vi "PIEZO_main.vi"() -> ()   [LabVIEW 2015]
uses:
  CONTROLS/Q_MCL_piezo_element.ctl
  CONTROLS/Q_main_element.ctl
  GLOBAL/Global_MCL_piezo.vi
  GLOBAL/Global_ABORT.vi
  GLOBAL/Global_MAIN.vi
  <vilib>/Utility/inputDevices.llb/keyboardAcquire.vi
  <vilib>/Utility/inputDevices.llb/closeKeyboard.vi
  <userlib>/Madlib.dll
  <vilib>/addons/control/pid/NI_PID_autopid.lvlib
panel:
  in  "Q_MCL_Piezo":T1
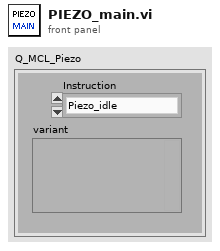
[diagram p1: front panel]
types:
  T1 = typedef "Q_MCL_piezo_element.ctl" = cluster{"variant":variant, "Instruction":enum16{"Piezo_idle", "Piezo_initialize", "Piezo_error", "Piezo_security_stop", "Piezo_read_z", "Piezo_move_z", "Piezo_keyboard_move", "Piezo_close_autofocus_calibration_ramp", "Piezo_change_init_state", "Piezo_init_autofocus", "Piezo_init_autofocus_merFISH_TL", "Piezo_autofocus", "Piezo_autofocus_merFISH_TL", "Piezo_stop_autofocus", "Piezo_stop_autofocus_merFISH_TL", "Piezo_autofocus_lost", "Piezo_resume_autofocus_merFISH_TL", "Piezo_check_z_position_merFISH_TL", "Piezo_init_ramp", "Piezo_move_z_ramp", "Piezo_close_ramp", "Piezo_close_merFISH", "Piezo_stop"}}
  T2 = cluster{"Setpoint":dbl, "Ref channel":bool, "dimension size":i32, "X_derivation":dbl[], "Y_derivation":dbl[], "Slope":dbl, "iteration":i32, "PID gains":cluster{"proportional gain (Kc)":dbl, "integral time (Ti, min)":dbl, "derivative time (Td, min)":dbl}, "z0":dbl, "Switch":bool, "Autocalibration":bool, "Init":bool, "i IR lost":i32, "Derivation array":dbl[], "QPDcount":u32}
  T3 = typedef "Q_main_element.ctl" = cluster{"variant":variant, "Instruction":enum16{"Main_idle", "Main_initialize", "Main_initialize_TDMS", "Main_initialize_Queue", "Main_error", "Main_DAQ_initialization_results", "Main_ASI_initialization_results", "Main_Piezo_initialization_results", "Main_Valve_initialization_results", "Main_Pump_initialization_results", "Main_CAMERA_initialization_results", "Main_FPGA_initialization_results", "Main_DAQ_error", "Main_ASI_error", "Main_Piezo_error", "Main_CAMERA_error", "Main_Valve_error", "Main_Pump_error", "Main_FPGA_error", "Main_start_acquiring", "Main_not_acquiring", "Main_acquiring", "Main_stop_acquiring", "Main_change_exposure", "Main_change_z_scan_parameters", "Main_define_ROI", "Main_define_mosaic", "Main_read_kinetic_time", "Main_cooler", "Main_read_temperature", "Main_save_XY", "Main_load_XY", "Main_discard_XY", "Main_move_to_XY", "Main_measure_QPD", "Main_autofocus_calibration", "Main_autofocus_initialization", "Main_autofocus_stop", "Main_save_PID", "Main_change_H_valve_position", "Main_two_way_valve", "Main_save_movie", "Main_init_single_scan", "Main_single_scan", "Main_stop_single_scan", "Main_merFISH_illumination_parameters", "Main_merFISH_buffer_probe_list", "Main_merFISH_injections_procedure", "Main_merFISH_save_setpoint", "Main_merFISH_DAPI_parameters", "Main_merFISH_Brightfield_parameters", "Main_merFISH_save_embryo_ROI", "Main_merFISH_init", "Main_merFISH_resume", "Main_merFISH_start_autofocus", "Main_merFISH_open_close_valve_merFISH", "Main_merFISH_open_close_valve_photobleaching", "Main_merFISH_hybridization", "Main_merFISH_move_to_ROI", "Main_merFISH_wait_stabilization", "Main_merFISH_move_to_REF", "Main_merFISH_scan", "Main_merFISH_photobleaching_injection", "Main_merFISH_photobleaching", "Main_merFISH_send_email", "Main_merFISH_close", "Main_STOP"}}
  T4 = enum16{"0", "1", "2", "3", "4", "5", "6", "7", "8", "9", "A", "B", "C", "D", "E", "F", "G", "H", "I", "J", "K", "L", "M", "N", "O", "P", "Q", "R", "S", "T", "U", "V", "W", "X", "Y", "Z", "F1", "F2", "F3", "F4", "F5", "F6", "F7", "F8", "F9", "F10", "F11", "F12", "F13", "F14", "F15", "ADD", "BACK", "BACKSLASH", "CAPITAL", "COMMA", "DECIMAL", "DELETE", "DIVIDE", "DOWN", "END", "EQUALS", "ESCAPE", "GRAVE (`)", "HOME", "INSERT", "LBRACKET", "LCONTROL", "LEFT", "L ALT", "LSHIFT", "LWIN", "MINUS", "MULTIPLY", "NEXT", "NUMLOCK", "NUMPAD_0", "NUMPAD_1", "NUMPAD_2", "NUMPAD_3", "NUMPAD_4", "NUMPAD_5", "NUMPAD_6", "NUMPAD_7", "NUMPAD_8", "NUMPAD_9", "PAUSE", "PERIOD", "PRIOR (PG UP)", "RBRACKET", "RCONTROL", "RETURN", "RIGHT", "R ALT", "RSHIFT", "RWIN", "SCROLL", "SEMICOLON", "SLASH", "SPACE", "SUBTRACT", "TAB", "UP", "ENTER (num pad)", "' (quote)"}
  T5 = cluster{"PID gains":cluster{"proportional gain (Kc)":dbl, "integral time (Ti, min)":dbl, "derivative time (Td, min)":dbl}, "QPD ref":cluster{"X":sgl, "Y":sgl, "SUM":sgl, "count":u32}}
  T6 = enum16{"Piezo_idle", "Piezo_initialize", "Piezo_error", "Piezo_security_stop", "Piezo_read_z", "Piezo_move_z", "Piezo_keyboard_move", "Piezo_close_autofocus_calibration_ramp", "Piezo_change_init_state", "Piezo_init_autofocus", "Piezo_init_autofocus_merFISH_TL", "Piezo_autofocus", "Piezo_autofocus_merFISH_TL", "Piezo_stop_autofocus", "Piezo_stop_autofocus_merFISH_TL", "Piezo_autofocus_lost", "Piezo_resume_autofocus_merFISH_TL", "Piezo_check_z_position_merFISH_TL", "Piezo_init_ramp", "Piezo_move_z_ramp", "Piezo_close_ramp", "Piezo_close_merFISH", "Piezo_stop"}
  T7 = enum16{"0", "1", "2", "3", "4", "5", "6", "7", "8", "9", "A", "B", "C", "D", "E", "F", "G", "H", "I", "J", "K", "L", "M", "N", "O", "P", "Q", "R", "S", "T", "U", "V", "W", "X", "Y", "Z", "F1", "F2", "F3", "F4", "F5", "F6", "F7", "F8", "F9", "F10", "F11", "F12", "F13", "F14", "F15", "ADD", "BACK", "BACKSLASH", "CAPITAL", "COMMA", "DECIMAL", "DELETE", "DIVIDE", "DOWN", "END", "EQUALS", "ESCAPE", "GRAVE (`)", "HOME", "INSERT", "LBRACKET", "LCONTROL", "LEFT", "L ALT", "LSHIFT", "LWIN", "MINUS", "MULTIPLY", "NEXT", "NUMLOCK", "NUMPAD_0", "NUMPAD_1", "NUMPAD_2", "NUMPAD_3", "NUMPAD_4", "NUMPAD_5", "NUMPAD_6", "NUMPAD_7", "NUMPAD_8", "NUMPAD_9", "PAUSE", "PERIOD", "PRIOR (PG UP)", "RBRACKET", "RCONTROL", "RETURN", "RIGHT", "R ALT", "RSHIFT", "RWIN", "SCROLL", "SEMICOLON", "SLASH", "SPACE", "SUBTRACT", "TAB", "UP", "ENTER (num pad)", "' (quote)"}[]
  T8 = cluster{"proportional gain (Kc)":dbl, "integral time (Ti, min)":dbl, "derivative time (Td, min)":dbl}
  T9 = cluster{"X":sgl, "Y":sgl, "SUM":sgl, "count":u32}
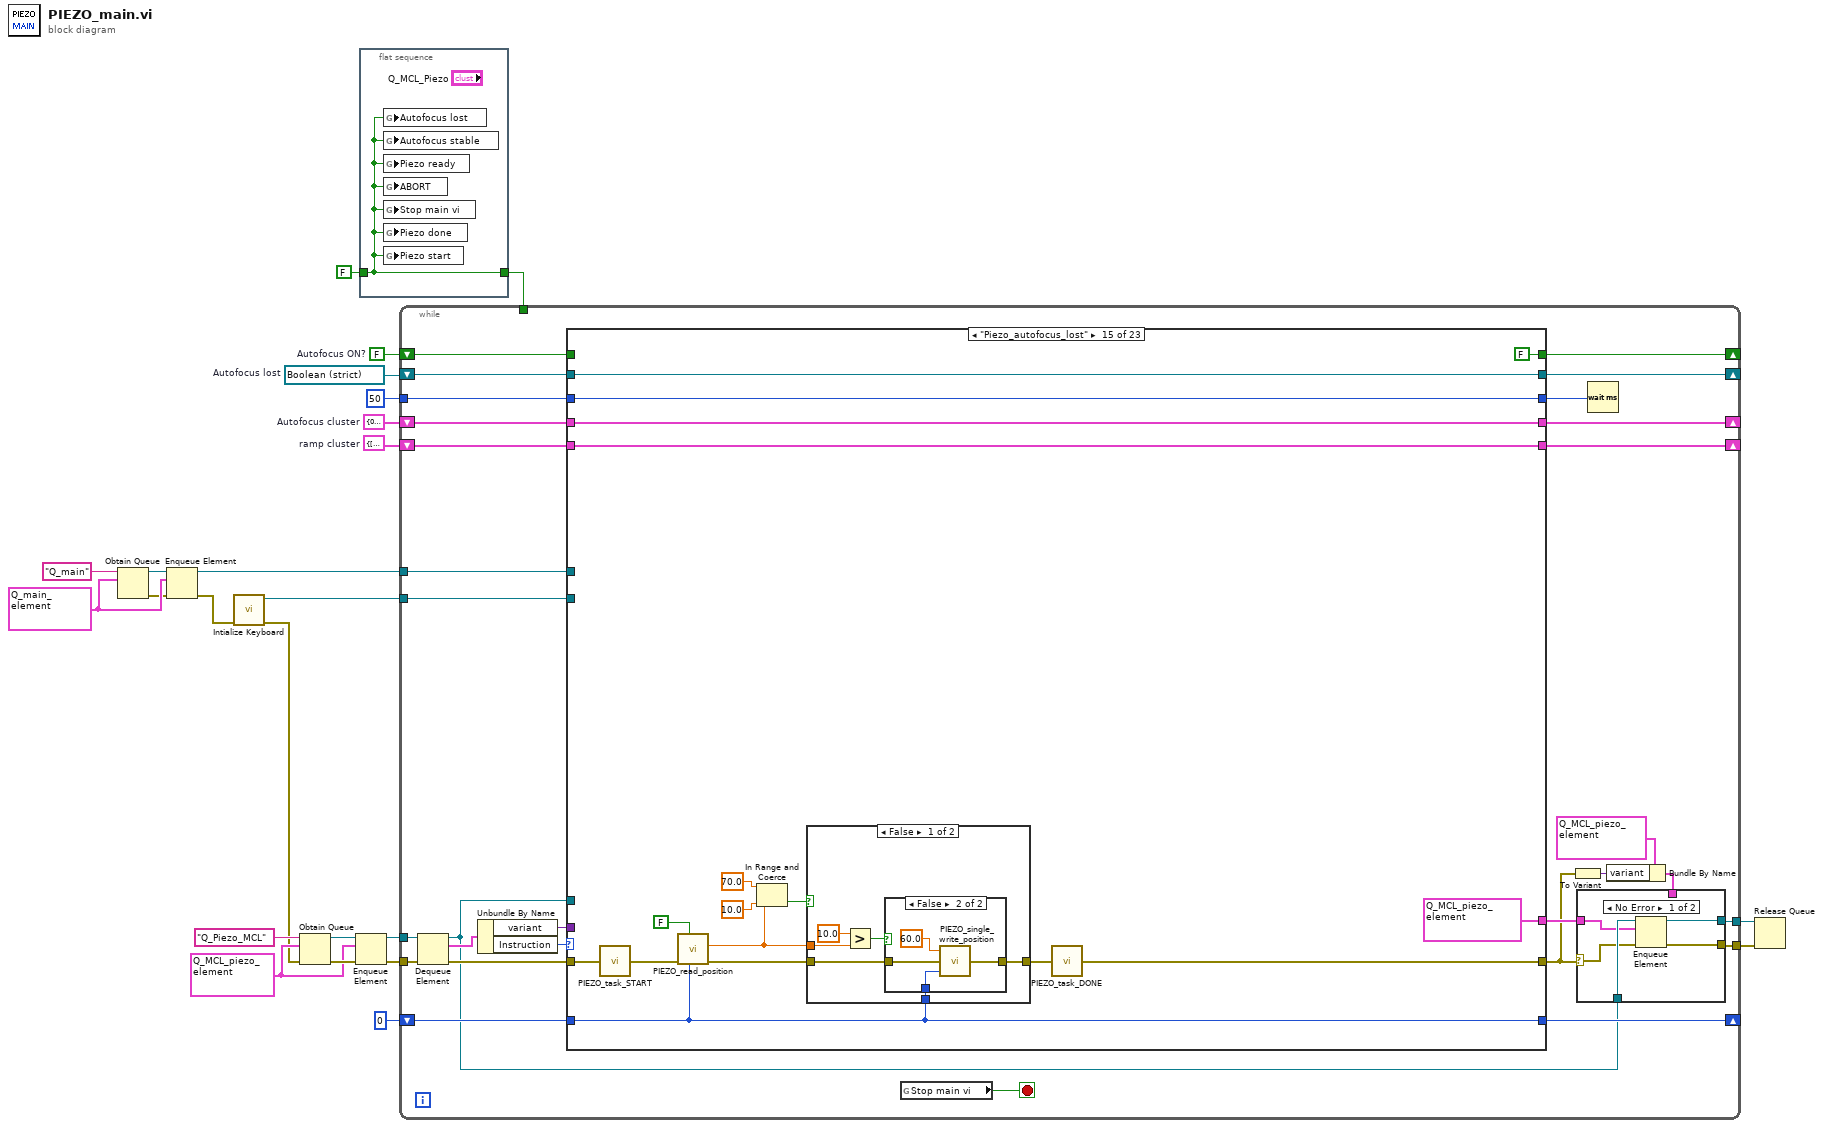
[diagram p0: block diagram]
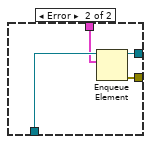
[diagram p2: hidden frame]
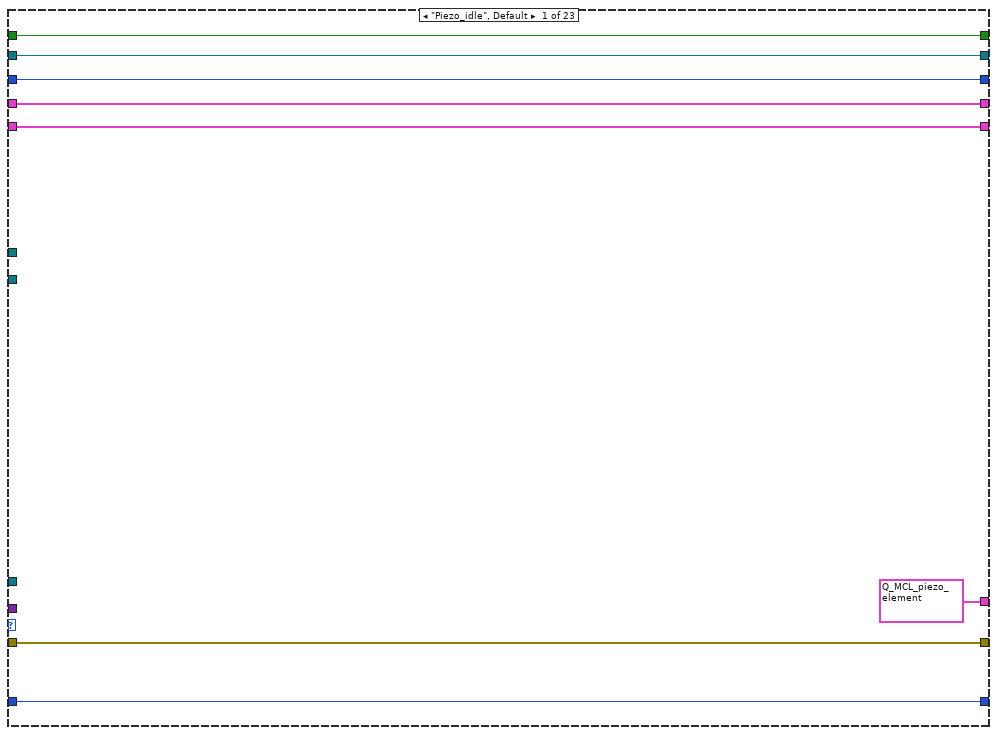
[diagram p3: hidden frame]
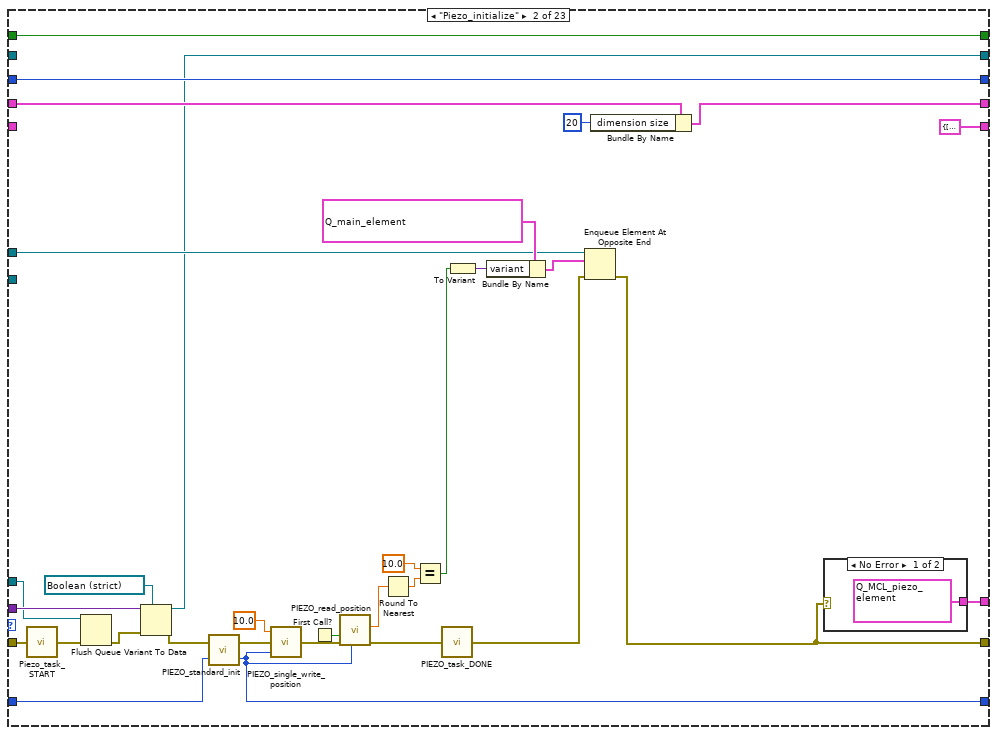
[diagram p4: hidden frame]
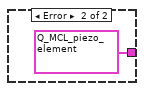
[diagram p5: hidden frame]
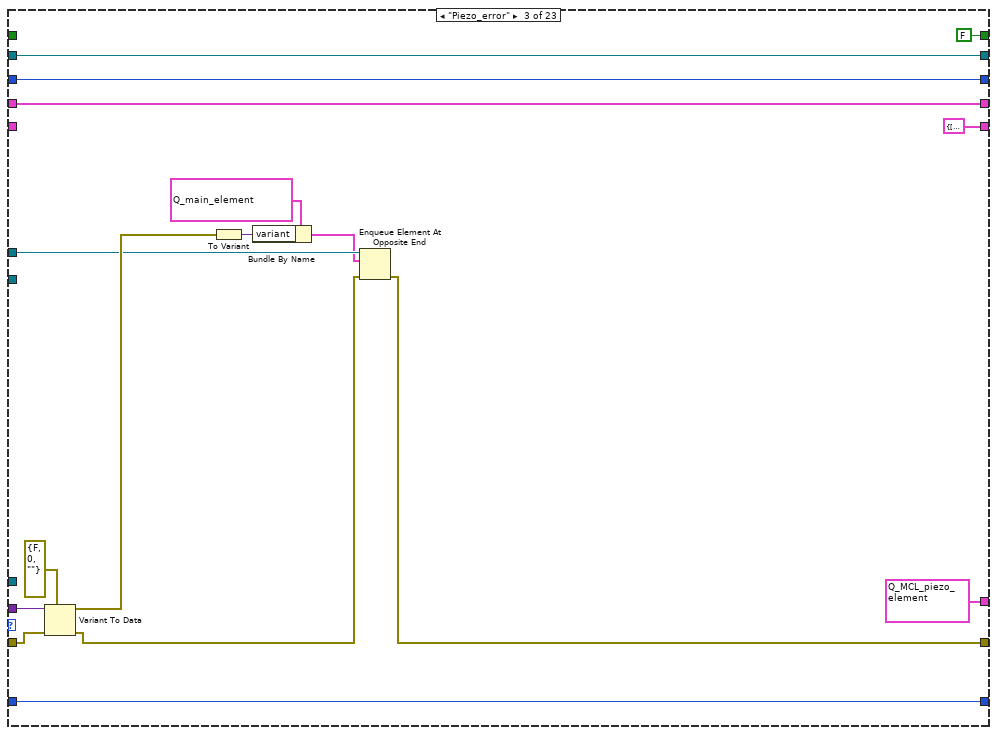
[diagram p6: hidden frame]
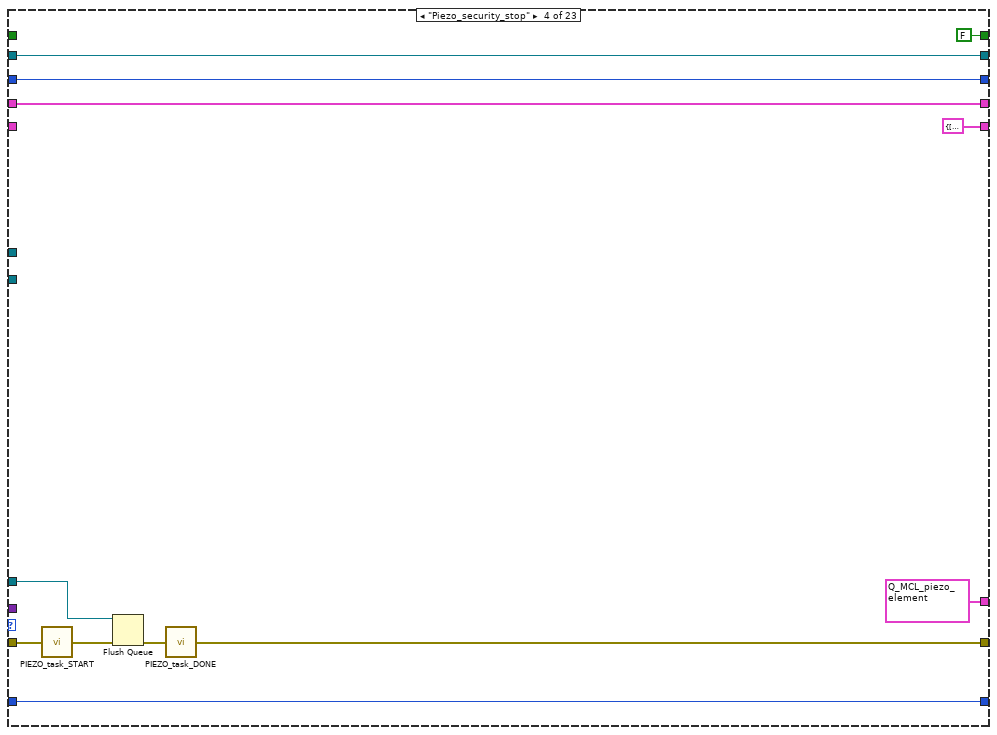
[diagram p7: hidden frame]
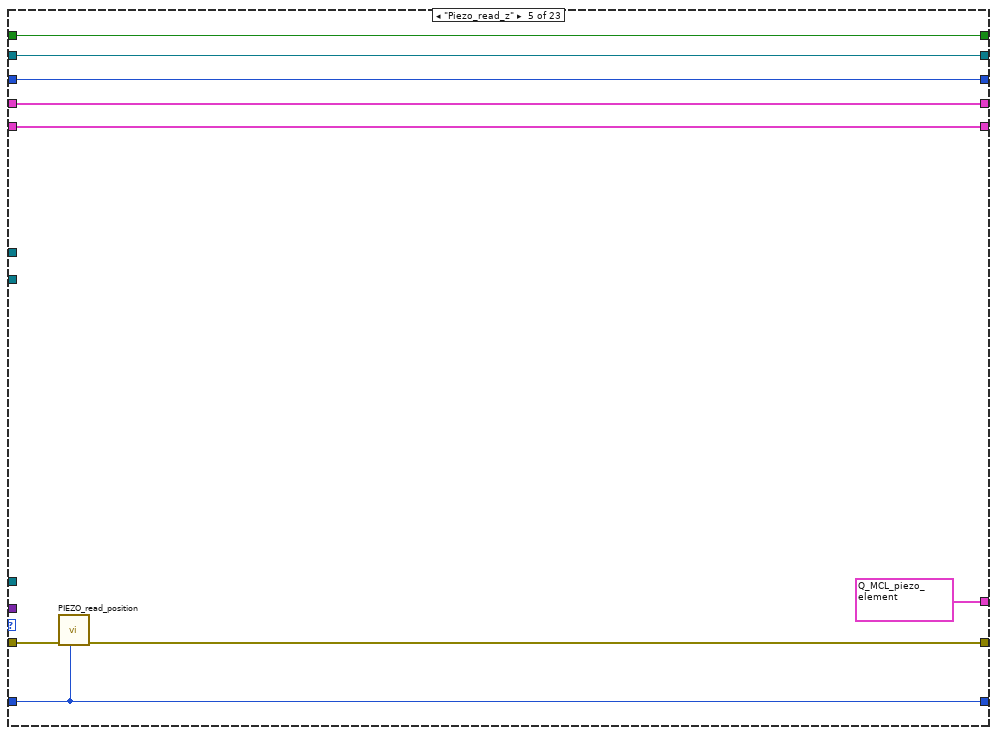
[diagram p8: hidden frame]
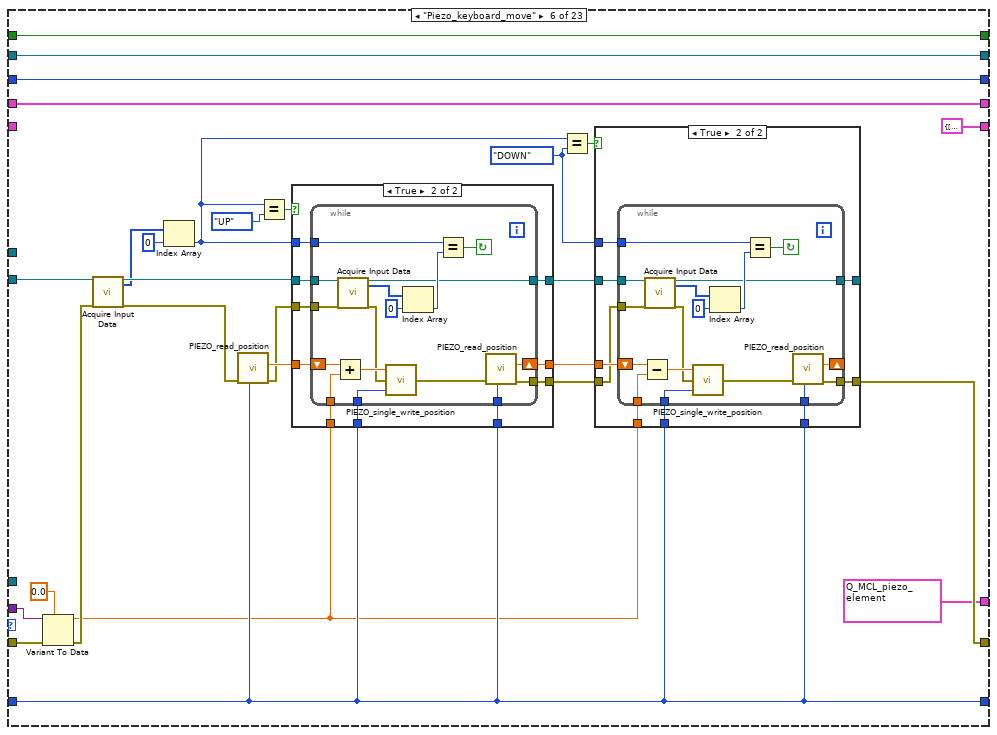
[diagram p9: hidden frame]
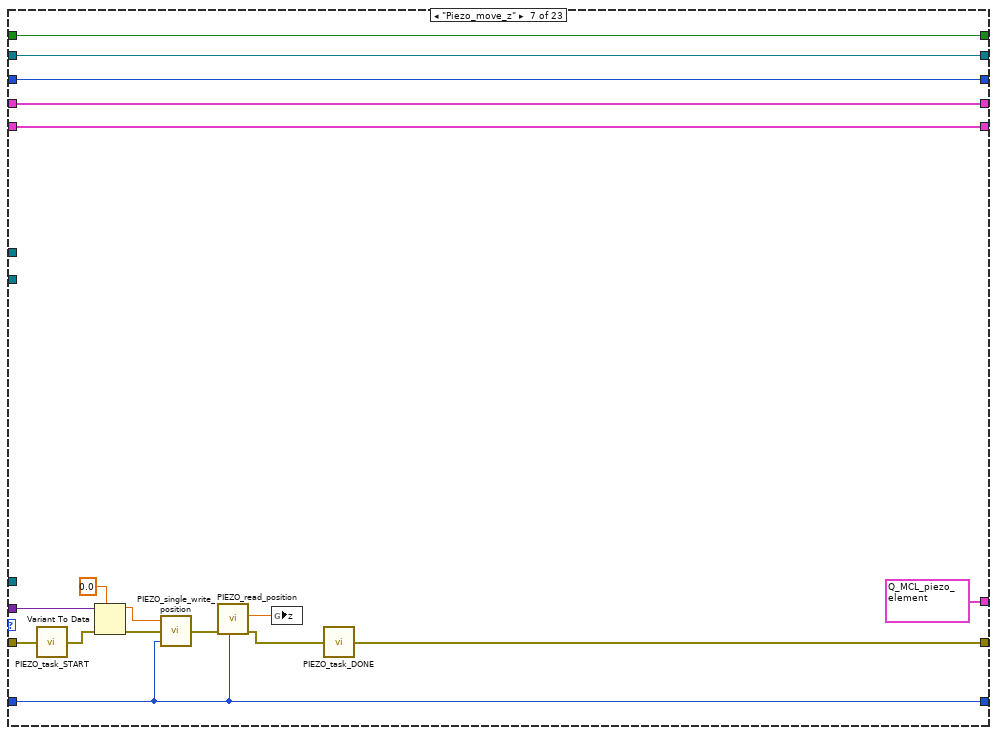
[diagram p12: hidden frame]
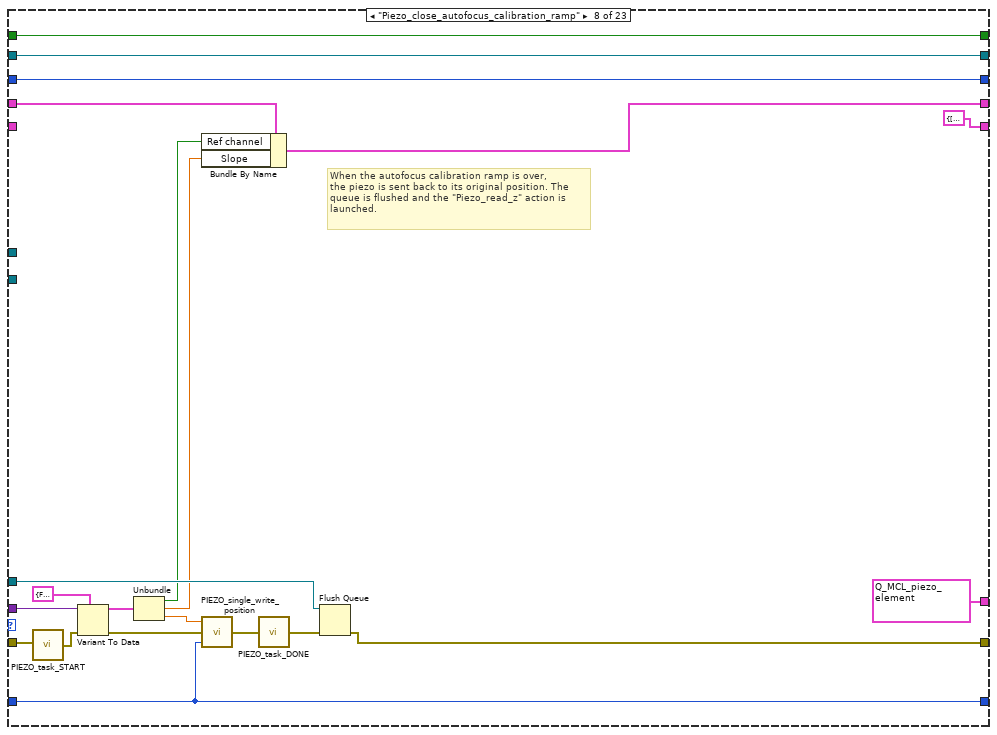
[diagram p13: hidden frame]
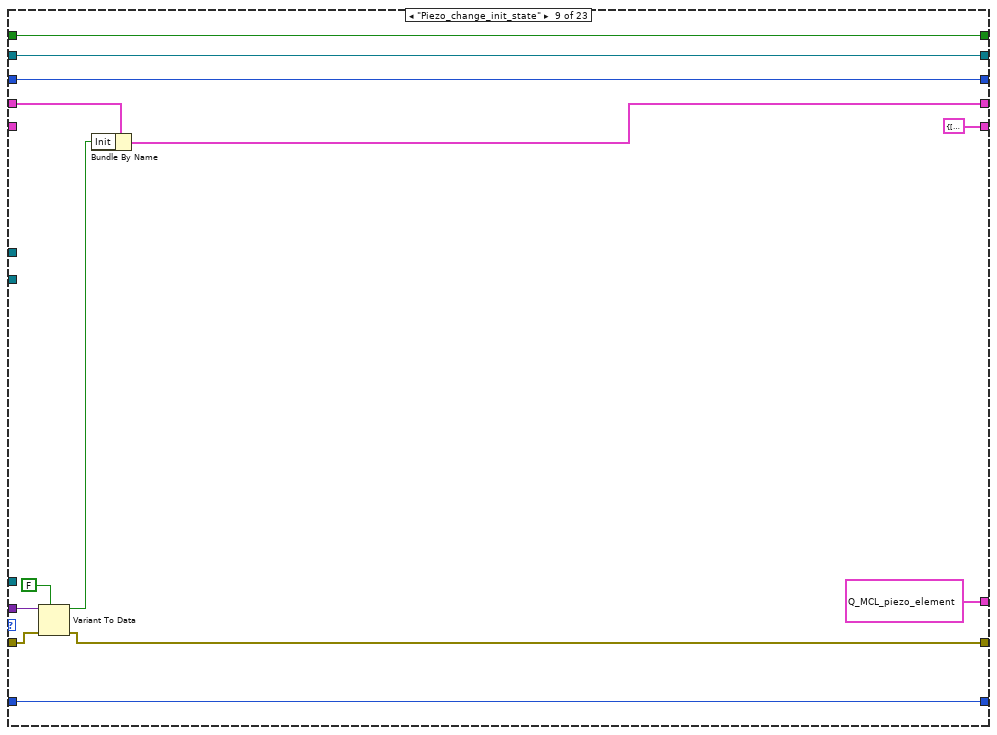
[diagram p14: hidden frame]
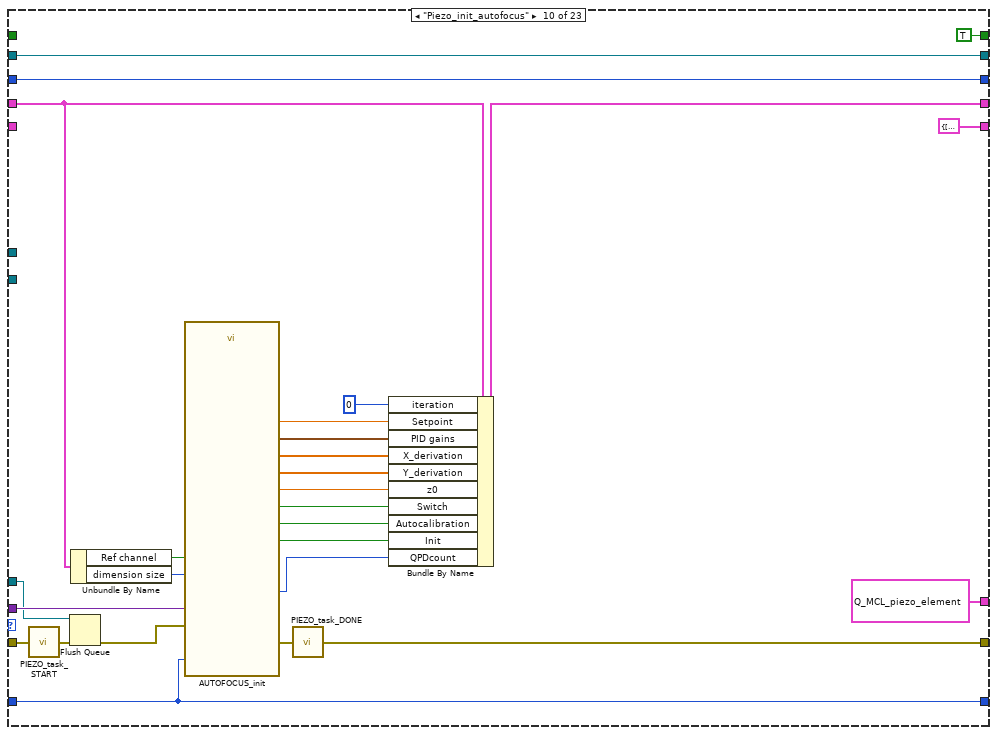
[diagram p15: hidden frame]
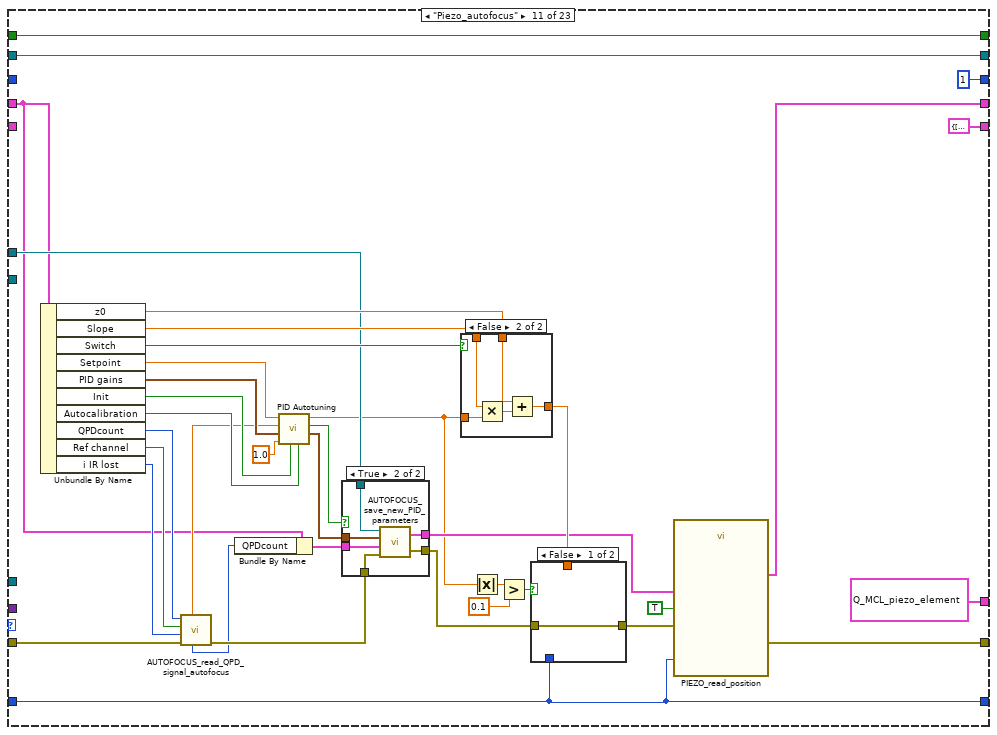
[diagram p16: hidden frame]
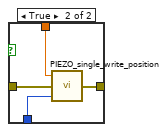
[diagram p17: hidden frame]
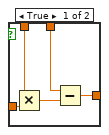
[diagram p19: hidden frame]
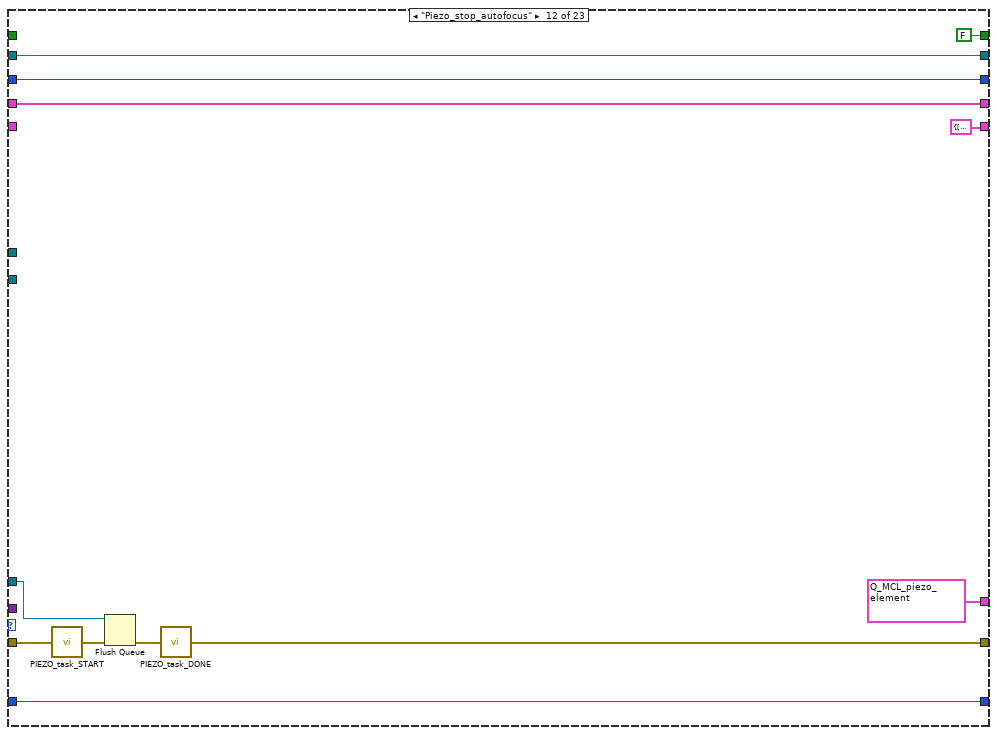
[diagram p20: hidden frame]
diagram:
  w1 = T2 {"Setpoint"=0.30117704117958327, "Ref channel"=TRUE, "dimension size"=20, "X_derivation"=[0.0, 0.1, 0.2, 0.3, 0.4, 0.5, 0.6, 0.7, 0.8, 0.9, 1.0, 1.1, 1.2, 1.3, 1.4, 1.5, 1.6, 1.7, 1.8, 1.9], "Y_derivation"=[24.741999437959365, 24.744723099615967, 24.751249609623358, 24.75114682993819, 24.745493947254644, 24.74472309961597, 24.73449652094301, 24.738145199766034, 24.731002011647725, 24.7278158414079, 24.736603504488706, 24.745956455837835, 24.74482587930113, 24.750787101040157, 24.75150655883624, 24.744106421505037, 24.74456893008824, 24.75294547442842, 24.75458994939091, 24.756799712621753], "Slope"=0.07279480071806545, "iteration"=1561, "PID gains"={"proportional gain (Kc)"=100.0, "integral time (Ti, min)"=0.05, "derivative time (Td, min)"=0.0}, "z0"=24.756799712621753, "Switch"=FALSE, "Autocalibration"=FALSE, "Init"=FALSE, "i IR lost"=0, "Derivation array"=[0.0167731809496238, 0.013820003755447539, 0.00923317051305809, 0.004692317656104263, 0.001858534908242838, 0.0003249538166207109, 0.0012101728342734128, 0.0028279869009538673, 0.0031819199521123664, 0.003610426233460469, 0.00491719651613391, 0.006489416587176226, 0.006445368150700671, 0.0068008467609944005, 0.006194214784715625, 0.004603834393355668, 0.004042410022944901, 0.004071389257482689, 0.004591083530175453, 0.004780028139339949], "QPDcount"=0}  # Autofocus cluster
  w2 = FALSE  # Autofocus ON?
  w3 = refnum<vi> refnum  # Autofocus lost
  w5 = cluster{"z positions":dbl[], "z0":dbl} {"z positions"=[], "z0"=0.0}  # ramp cluster
  w11 = T1 {"variant"=variant, "Instruction"=enum."Piezo_idle"} ("Q_MCL_Piezo")
  w17 = T3 {"variant"=variant, "Instruction"=enum."Main_idle"} ("Q_main_element")
  n1 = Obtain Queue(name (unnamed)="Q_main", element data type=w17) -> (queue out=w15:refnum<queue>, error out=w16:errorcluster)  [unwired: 3 in, 1 out]
  n2 = Enqueue Element(queue=w15, element=w17, error in (no error)=w16) -> (queue out=w13:refnum<queue>, error out=w8:errorcluster)  [unwired: 1 in, 1 out]
  n3 = call <vilib>:"Intialize Keyboard.vi"("error in (no error)"=w8) -> ("error out"=w7:errorcluster, "device ID"=w6:refnum<k1>)  [unwired: 9 in]
  n4 = Obtain Queue(name (unnamed)="Q_Piezo_MCL", element data type=w11, error in (no error)=w7) -> (queue out=w23:refnum<queue>, error out=w22:errorcluster)  [unwired: 2 in, 1 out]
  n5 = Enqueue Element(queue=w23, element=w11, error in (no error)=w22) -> (queue out=w21:refnum<queue>, error out=w20:errorcluster)  [unwired: 1 in, 1 out]
  n6 = flat-sequence {
    tunnel: FALSE ("Stop main vi") -> [w25]
    tunnel: [w25] -> w10
    frame #0 {
      n7 = global write "Global_MCL_piezo.vi" "Autofocus lost"(w25) -> ()
      n8 = global write "Global_MCL_piezo.vi" "Autofocus stable"(w25) -> ()
      n9 = global write "Global_MCL_piezo.vi" "Piezo ready"(w25) -> ()
      n10 = global write "Global_ABORT.vi" "ABORT"(w25) -> ()
      n11 = global write "Global_MAIN.vi" "Stop main vi"(w25) -> ()
      n12 = global write "Global_MCL_piezo.vi" "Piezo done"(w25) -> ()
      n13 = global write "Global_MCL_piezo.vi" "Piezo start"(w25) -> ()
    }
  }
  n14 = while {
    tunnel: w21 -> [w53]
    tunnel: w20 -> [w31]
    tunnel: [w48] -> w19
    tunnel: [w47] -> w18
    tunnel: w13 -> [w46]
    tunnel: w10 -> [_]
    shift-right: [w43] -> _
    shift-left: 0 ("Incoming Handle") -> [w44]
    tunnel: w6 -> [w42]
    shift-right: [w36] -> _
    shift-left: w1 -> [w37]
    shift-right: [w34] -> _
    shift-left: w5 -> [w35]
    tunnel: u32 50 ("milliseconds to wait") -> [w33]
    shift-right: [w29] -> _
    shift-left: w3 -> [w30]
    shift-right: [w27] -> _
    shift-left: w2 -> [w28]
    stop <- w54 stop-if-true
    n15 = Dequeue Element(queue=w53, error in (no error)=w31) -> (queue out=w26:refnum<queue>, element=w52:T1, error out=w50:errorcluster)  [unwired: 1 in, 1 out]
    n16 = Unbundle By Name(w52) -> ("variant"=w45:variant, "Instruction"=w51:T6)
    n17 = case shown="\"Piezo_autofocus_lost\"" w51 {
      tunnel: w50 -> [w71 w103 w120 w134 w143 w154 w246 w267 w273 w305 w325 w371 w408 w421 w512 w553 w616 w621 w646 w674 w706 w718 w739]
      tunnel: [w71 w83 w108 w131 w142 w155 w236 w259 w270 w281 w324 w368 w389 w433 w498 w540 w612 w620 w643 w667 w704 w716 w729] -> w39
      tunnel: [T1 {"variant"=variant, "Instruction"=enum."Piezo_idle"} ("Q_MCL_Piezo") w102 T1 {"variant"=variant, "Instruction"=enum."Piezo_idle"} ("Q_MCL_Piezo") T1 {"variant"=variant, "Instruction"=enum."Piezo_idle"} ("Q_MCL_Piezo") T1 {"variant"=variant, "Instruction"=enum."Piezo_read_z"} ("Q_MCL_Piezo") T1 {"variant"=variant, "Instruction"=enum."Piezo_read_z"} ("Q_MCL_Piezo") T1 {"variant"=variant, "Instruction"=enum."Piezo_idle"} ("Q_MCL_Piezo") T1 {"variant"=variant, "Instruction"=enum."Piezo_read_z"} ("Q_MCL_Piezo") T1 {"variant"=variant, "Instruction"=enum."Piezo_autofocus"} ("Q_MCL_Piezo") T1 {"variant"=variant, "Instruction"=enum."Piezo_autofocus"} ("Q_MCL_Piezo") T1 {"variant"=variant, "Instruction"=enum."Piezo_autofocus"} ("Q_MCL_Piezo") T1 {"variant"=variant, "Instruction"=enum."Piezo_read_z"} ("Q_MCL_Piezo") T1 {"variant"=variant, "Instruction"=enum."Piezo_autofocus_merFISH_TL"} ("Q_MCL_Piezo") w441 T1 {"variant"=variant, "Instruction"=enum."Piezo_read_z"} ("Q_MCL_Piezo") w544 w610 T1 {"variant"=variant, "Instruction"=enum."Piezo_read_z"} ("Q_MCL_Piezo") T1 {"variant"=variant, "Instruction"=enum."Piezo_idle"} ("Q_MCL_Piezo") T1 {"variant"=variant, "Instruction"=enum."Piezo_idle"} ("Q_MCL_Piezo") T1 {"variant"=variant, "Instruction"=enum."Piezo_read_z"} ("Q_MCL_Piezo") T1 {"variant"=variant, "Instruction"=enum."Piezo_read_z"} ("Q_MCL_Piezo") T1 {"variant"=variant, "Instruction"=enum."Piezo_idle"} ("Q_MCL_Piezo")] -> w49
      tunnel: w46 -> [_ w94 w114 _ _ _ _ _ _ _ w337 _ _ _ _ _ _ _ _ _ _ _ _]
      tunnel: w45 -> [_ w82 w121 _ _ w153 w245 w266 w280 w304 _ _ w403 _ _ _ _ _ _ w673 w702 _ _]
      tunnel: w26 -> [_ w74 _ w132 _ _ _ w258 _ w287 _ w378 w404 _ _ w528 _ w619 w632 _ _ w723 w731]
      tunnel: w44 -> [w69 w101 w122 w130 w140 w156 w239 w263 w279 w290 w342 w379 w396 w429 w499 w542 w613 w630 w645 w669 w692 w724 w740]
      tunnel: [w69 w88 w122 w130 w140 w156 w239 w263 w279 w290 w342 w379 w396 w429 w499 w542 w613 w630 w645 w669 w692 w724 w740] -> w43
      tunnel: w42 -> [_ _ _ _ _ w164 _ _ _ _ _ _ _ _ _ _ _ _ _ _ _ _ w737]
      tunnel: w37 -> [w68 w80 w111 w128 w139 w151 w234 w254 w277 w303 w315 w376 w407 w432 w507 w547 w607 w628 w642 w665 w703 w721 w735]
      tunnel: [w68 w79 w111 w128 w139 w151 w234 w252 w276 w306 w334 w376 w409 w431 w507 w531 w607 w628 w642 w665 w703 w721 w735] -> w36
      tunnel: w35 -> [w67 _ _ _ w138 _ w233 _ _ _ _ _ _ _ w504 _ _ _ w639 w656 w690 _ _]
      tunnel: [w67 cluster{"z positions":dbl[], "z0":dbl} {"z positions"=[], "z0"=0.0} ("ramp cluster") cluster{"z positions":dbl[], "z0":dbl} {"z positions"=[], "z0"=0.0} ("ramp cluster") cluster{"z positions":dbl[], "z0":dbl} {"z positions"=[], "z0"=0.0} ("ramp cluster") w138 cluster{"z positions":dbl[], "z0":dbl} {"z positions"=[], "z0"=0.0} ("ramp cluster") w233 cluster{"z positions":dbl[], "z0":dbl} {"z positions"=[], "z0"=0.0} ("ramp cluster") cluster{"z positions":dbl[], "z0":dbl} {"z positions"=[], "z0"=0.0} ("ramp cluster") cluster{"z positions":dbl[], "z0":dbl} {"z positions"=[], "z0"=0.0} ("ramp cluster") cluster{"z positions":dbl[], "z0":dbl} {"z positions"=[], "z0"=0.0} ("ramp cluster") cluster{"z positions":dbl[], "z0":dbl} {"z positions"=[], "z0"=0.0} ("ramp cluster") cluster{"z positions":dbl[], "z0":dbl} {"z positions"=[], "z0"=0.0} ("ramp cluster") w435 w504 cluster{"z positions":dbl[], "z0":dbl} {"z positions"=[], "z0"=0.0} ("ramp cluster") cluster{"z positions":dbl[], "z0":dbl} {"z positions"=[], "z0"=0.0} ("ramp cluster") cluster{"z positions":dbl[], "z0":dbl} {"z positions"=[], "z0"=0.0} ("ramp cluster") w638 w654 w689 cluster{"z positions":dbl[], "z0":dbl} {"z positions"=[], "z0"=0.0} ("ramp cluster") cluster{"z positions":dbl[], "z0":dbl} {"z positions"=[], "z0"=0.0} ("ramp cluster")] -> w34
      tunnel: w33 -> [w66 w84 w109 w126 w137 w149 w232 w249 w274 w289 _ w374 w405 _ w506 _ _ w626 _ w653 _ w719 w733]
      tunnel: [w66 w84 w109 w126 w137 w149 w232 w249 w274 w289 u32 1 ("milliseconds to wait") w374 w405 u32 1 ("milliseconds to wait") w506 u32 1 ("milliseconds to wait") u32 1 ("milliseconds to wait") w626 u32 1 ("milliseconds to wait") w653 u32 50 ("milliseconds to wait") w719 w733] -> w32
      tunnel: w30 -> [w65 _ w107 w124 w136 w145 w231 w248 w269 w285 w322 w373 w387 w428 w505 w535 w611 w625 w636 w652 w687 w713 w728]
      tunnel: [w65 w72 w107 w124 w136 w145 w231 w248 w269 w285 w322 w373 w387 w428 w505 w535 w611 w625 w636 w652 w687 w713 w728] -> w29
      tunnel: w28 -> [w64 w78 _ _ w135 w144 w230 w247 w268 _ w319 _ _ w422 _ _ w605 _ w635 w651 w686 w712 w727]
      tunnel: [w64 w78 FALSE ("Autofocus ON?") FALSE ("Autofocus ON?") w135 w144 w230 w247 w268 TRUE ("Autofocus ON?") w319 FALSE ("Autofocus ON?") TRUE ("Autofocus ON?") w422 FALSE ("Autofocus ON?") w534 w605 FALSE ("Autofocus ON?") w635 w651 w686 w712 w727] -> w27
      frame "Piezo_idle", Default {
      }
      frame "Piezo_initialize" {
        n18 = call "Piezo_task_START.vi"("error in"=w103) -> ("error out"=w77:errorcluster)
        n19 = Flush Queue(queue=w74, error in (no error)=w77) -> (error out=w76:errorcluster)  [unwired: 2 out]
        n20 = Variant To Data(error in=w76, type=refnum<vi> refnum ("Autofocus lost Refnum"), Variant=w82) -> (data=w72:refnum<vi>, error out=w75:errorcluster)
        n21 = call "PIEZO_standard_init.vi"("Incoming Handle"=w101, "error in"=w75) -> ("Outgoing Handle"=w88:i32, "error out"=w89:errorcluster)
        n22 = call "PIEZO_single_write_position.vi"("handle"=w88, "error in"=w89, "Zposition setpoint"=10.0) -> ("error out"=w86:errorcluster)  [unwired: 2 in]
        n23 = First Call?() -> (First Call?: T/F=w90:bool)
        n24 = call "PIEZO_read_position.vi"("MCL Handle"=w88, "error MCL in"=w86, "Reset"=w90) -> ("error MCL out"=w100:errorcluster, "Z piezo"=w92:dbl)  [unwired: 5 in, 2 out]
        n25 = Round To Nearest(number=w92) -> (nearest integer value=w99:dbl)
        n26 = Equal?(x=10.0 ("Zposition setpoint"), y=w99) -> (x = y?=w91:bool)
        n27 = call "PIEZO_task_DONE.vi"("error in"=w100) -> ("error out"=w93:errorcluster)
        n28 = To Variant(anything=w91) -> (Variant=w96:variant)
        n29 = Bundle By Name(cluster=T3 {"variant"=variant, "Instruction"=enum."Main_Piezo_initialization_results"} ("element"), "variant"=w96) -> (w97:T3)
        n30 = Enqueue Element At Opposite End(queue=w94, element=w97, error in (no error)=w93) -> (error out=w83:errorcluster)  [unwired: 1 in, 2 out]
        n31 = Bundle By Name(cluster=w80, "dimension size"=20) -> (w79:T2)
        n32 = case shown="No Error" w83 {
          tunnel: [T1 {"variant"=variant, "Instruction"=enum."Piezo_read_z"} ("Q_MCL_Piezo") T1 {"variant"=variant, "Instruction"=enum."Piezo_idle"} ("Q_MCL_Piezo")] -> w102
          frame No Error {
          }
          frame Error {
          }
        }
      }
      frame "Piezo_error" {
        n33 = Variant To Data(error in=w120, type=errorcluster {"status"=FALSE, "code"=0, "source"=""} ("error out"), Variant=w121) -> (data=w115:errorcluster, error out=w112:errorcluster)
        n34 = To Variant(anything=w115) -> (Variant=w116:variant)
        n35 = Bundle By Name(cluster=T3 {"variant"=variant, "Instruction"=enum."Main_Piezo_error"} ("Q_main_element"), "variant"=w116) -> (w113:T3)
        n36 = Enqueue Element At Opposite End(queue=w114, element=w113, error in (no error)=w112) -> (error out=w108:errorcluster)  [unwired: 1 in, 2 out]
      }
      frame "Piezo_security_stop" {
        n37 = call "PIEZO_task_START.vi"("error in"=w134) -> ("error out"=w133:errorcluster)
        n38 = Flush Queue(queue=w132, error in (no error)=w133) -> (error out=w125:errorcluster)  [unwired: 2 out]
        n39 = call "PIEZO_task_DONE.vi"("error in"=w125) -> ("error out"=w131:errorcluster)
      }
      frame "Piezo_read_z" {
        n40 = call "PIEZO_read_position.vi"("MCL Handle"=w140, "error MCL in"=w143) -> ("error MCL out"=w142:errorcluster)  [unwired: 6 in, 3 out]
      }
      frame "Piezo_keyboard_move" {
        w157 = T4."DOWN" ("x")
        n41 = Variant To Data(error in=w154, type=0.0 ("Piezo step (um)"), Variant=w153) -> (data=w146:dbl, error out=w152:errorcluster)
        n42 = call-poly <vilib>:"Acquire Input Data.vi"("device ID"=w164, "error in (no error)"=w152) -> ("device ID"=w169:refnum<k1>, "keys pressed"=w165:T7, "error out"=w167:errorcluster)  [unwired: 15 in]
        n43 = Index Array(array=w165, index=0) -> (element=w161:T4)
        n44 = call "PIEZO_read_position.vi"("MCL Handle"=w156, "error MCL in"=w167) -> ("error MCL out"=w170:errorcluster, "Z piezo"=w171:dbl)  [unwired: 6 in, 2 out]
        n45 = Equal?(x=w161, y=T4."UP" ("x")) -> (x = y?=w163:bool)
        n46 = case shown="True" w163 {
          tunnel: w169 -> [w201 w212]
          tunnel: w170 -> [w202 w211]
          tunnel: w161 -> [_ w210]
          tunnel: w171 -> [w200 w209]
          tunnel: w146 -> [_ w208]
          tunnel: [w202 w204] -> w158
          tunnel: [w201 w207] -> w160
          tunnel: w156 -> [_ w206]
          tunnel: w156 -> [_ w205]
          tunnel: [w200 w203] -> w159
          frame False {
          }
          frame True {
            n47 = while {
              tunnel: w212 -> [w227]
              tunnel: w211 -> [w226]
              tunnel: w210 -> [w225]
              shift-right: [w215] -> w203
              shift-left: w209 -> [w223]
              tunnel: w208 -> [w222]
              tunnel: [w221] -> w207
              tunnel: w206 -> [w219]
              tunnel: w205 -> [w216]
              tunnel: [w214] -> w204
              stop <- w213 continue-if-true
              n48 = Add(x=w223, y=w222) -> (x+y=w220:dbl)
              n49 = call-poly <vilib>:"Acquire Input Data.vi"("device ID"=w227, "error in (no error)"=w226) -> ("device ID"=w221:refnum<k1>, "keys pressed"=w228:T7, "error out"=w218:errorcluster)  [unwired: 15 in]
              n50 = call "PIEZO_single_write_position.vi"("handle"=w219, "error in"=w218, "Zposition setpoint"=w220) -> ("error out"=w217:errorcluster)  [unwired: 2 in]
              n51 = Index Array(array=w228, index=0) -> (element=w224:T4)
              n52 = Equal?(x=w225, y=w224) -> (x = y?=w213:bool)
              n53 = call "PIEZO_read_position.vi"("MCL Handle"=w216, "error MCL in"=w217) -> ("error MCL out"=w214:errorcluster, "Z piezo"=w215:dbl)  [unwired: 6 in, 2 out]
            }
          }
        }
        n54 = Equal?(x=w161, y=w157) -> (x = y?=w162:bool)
        n55 = case shown="True" w162 {
          tunnel: w160 -> [w173 w182]
          tunnel: w157 -> [_ w181]
          tunnel: w159 -> [_ w180]
          tunnel: w146 -> [_ w179]
          tunnel: [w172 w175] -> w155
          tunnel: [w173 w178] -> _
          tunnel: w156 -> [_ w177]
          tunnel: w156 -> [_ w176]
          tunnel: w158 -> [w172 w174]
          frame False {
          }
          frame True {
            n56 = while {
              tunnel: w182 -> [w197]
              tunnel: w174 -> [w196]
              tunnel: w181 -> [w195]
              shift-right: [w185] -> _
              shift-left: w180 -> [w193]
              tunnel: w179 -> [w192]
              tunnel: [w191] -> w178
              tunnel: w177 -> [w189]
              tunnel: w176 -> [w186]
              tunnel: [w184] -> w175
              stop <- w183 continue-if-true
              n57 = Subtract(x=w193, y=w192) -> (x-y=w190:dbl)
              n58 = call-poly <vilib>:"Acquire Input Data.vi"("device ID"=w197, "error in (no error)"=w196) -> ("device ID"=w191:refnum<k1>, "keys pressed"=w198:T7, "error out"=w188:errorcluster)  [unwired: 15 in]
              n59 = call "PIEZO_single_write_position.vi"("handle"=w189, "error in"=w188, "Zposition setpoint"=w190) -> ("error out"=w187:errorcluster)  [unwired: 2 in]
              n60 = Index Array(array=w198, index=0) -> (element=w194:T4)
              n61 = Equal?(x=w195, y=w194) -> (x = y?=w183:bool)
              n62 = call "PIEZO_read_position.vi"("MCL Handle"=w186, "error MCL in"=w187) -> ("error MCL out"=w184:errorcluster, "Z piezo"=w185:dbl)  [unwired: 6 in, 2 out]
            }
          }
        }
      }
      frame "Piezo_move_z" {
        n63 = call "PIEZO_task_START.vi"("error in"=w246) -> ("error out"=w244:errorcluster)
        n64 = Variant To Data(error in=w244, type=0.0 ("Z"), Variant=w245) -> (data=w241:dbl, error out=w242:errorcluster)
        n65 = call "PIEZO_single_write_position.vi"("handle"=w239, "error in"=w242, "Zposition setpoint"=w241) -> ("error out"=w240:errorcluster)  [unwired: 2 in]
        n66 = call "PIEZO_read_position.vi"("MCL Handle"=w239, "error MCL in"=w240) -> ("error MCL out"=w237:errorcluster, "Z piezo"=w238:dbl)  [unwired: 6 in, 2 out]
        n67 = global write "Global_MCL_piezo.vi" "z"(w238) -> ()
        n68 = call "PIEZO_task_DONE.vi"("error in"=w237) -> ("error out"=w236:errorcluster)
      }
      frame "Piezo_close_autofocus_calibration_ramp" {
        # "When the autofocus calibration ramp is over,\nthe piezo is sent back to its original position. The \nqueue is flushed and the \"Piezo_read_z\" action is \nlaunched."
        n69 = call "PIEZO_task_START.vi"("error in"=w267) -> ("error out"=w265:errorcluster)
        n70 = Variant To Data(error in=w265, type=cluster{"Channel":bool, "slope":dbl, "z0":dbl} {"Channel"=FALSE, "slope"=0.0, "z0"=0.0} ("output cluster"), Variant=w266) -> (data=w257:cluster{"Channel":bool, "slope":dbl, "z0":dbl}, error out=w264:errorcluster)
        n71 = Unbundle(w257) -> ("Channel"=w251:bool, "slope"=w253:dbl, "z0"=w256:dbl)
        n72 = Bundle By Name(cluster=w254, "Ref channel"=w251, "Slope"=w253) -> (w252:T2)
        n73 = call "PIEZO_single_write_position.vi"("handle"=w263, "error in"=w264, "Zposition setpoint"=w256) -> ("error out"=w262:errorcluster)  [unwired: 2 in]
        n74 = call "PIEZO_task_DONE.vi"("error in"=w262) -> ("error out"=w260:errorcluster)
        n75 = Flush Queue(queue=w258, error in (no error)=w260) -> (error out=w259:errorcluster)  [unwired: 2 out]
      }
      frame "Piezo_change_init_state" {
        n76 = Variant To Data(error in=w273, type=FALSE, Variant=w280) -> (data=w271:bool, error out=w270:errorcluster)
        n77 = Bundle By Name(cluster=w277, "Init"=w271) -> (w276:T2)
      }
      frame "Piezo_init_autofocus" {
        n78 = call "PIEZO_task_START.vi"("error in"=w305) -> ("error out"=w282:errorcluster)
        n79 = Flush Queue(queue=w287, error in (no error)=w282) -> (error out=w288:errorcluster)  [unwired: 2 out]
        n80 = Unbundle By Name(w303) -> ("Ref channel"=w301:bool, "dimension size"=w302:i32)
        n81 = call "AUTOFOCUS_init.vi"("variant"=w304, "Dimension size"=w302, "MCL Handle"=w290, "channel"=w301, "error in"=w288) -> ("Init"=w286:bool, "Y initialized array"=w299:dbl[], "X initialized array"=w298:dbl[], "Z0"=w300:dbl, "Autotune"=w292:bool, "Setpoint"=w296:dbl, "Switch"=w294:bool, "QPDcount OUT"=w283:u32, "PID cluster"=w297:T8, "error out"=w293:errorcluster)  [unwired: 1 in]
        n82 = call "PIEZO_task_DONE.vi"("error in"=w293) -> ("error out"=w281:errorcluster)
        n83 = Bundle By Name(cluster=w303, "iteration"=0, "Setpoint"=w296, "PID gains"=w297, "X_derivation"=w298, "Y_derivation"=w299, "z0"=w300, "Switch"=w294, "Autocalibration"=w292, "Init"=w286, "QPDcount"=w283) -> (w306:T2)
      }
      frame "Piezo_autofocus" {
        n84 = Unbundle By Name(w315) -> ("z0"=w340:dbl, "Slope"=w339:dbl, "Switch"=w338:bool, "Setpoint"=w330:dbl, "PID gains"=w329:T8, "Init"=w327:bool, "Autocalibration"=w328:bool, "QPDcount"=w316:u32, "Ref channel"=w317:bool, "i IR lost"=w318:i32)
        n85 = call "AUTOFOCUS_read_QPD_signal_autofocus.vi"("error in"=w325, "i IR lost"=w318, "channel"=w317, "QPDcount"=w316) -> ("error out"=w326:errorcluster, "QPDcount OUT"=w313:u32, "QPD"=w321:dbl)  [unwired: 1 in, 2 out]
        n86 = Bundle By Name(cluster=w315, "QPDcount"=w313) -> (w314:T2)
        n87 = call <vilib>:"PID Autotuning.vi"("autotune? (F)"=w328, "reinitialize? (F)"=w327, "dt (s)"=1.0, "PID gains"=w329, "process variable"=w321, "setpoint"=w330) -> ("PID gains out"=w331:T8, "tuning completed?"=w332:bool, "output"=w310:dbl)  [unwired: 2 in, 1 out]
        n88 = case shown="True" w332 {
          tunnel: w331 -> [_ w356]
          tunnel: w314 -> [w350 w352]
          tunnel: w326 -> [w351 w357]
          tunnel: w337 -> [_ w355]
          tunnel: [w351 w354] -> w308
          tunnel: [w350 w353] -> w320
          frame False {
          }
          frame True {
            n89 = call "AUTOFOCUS_save_new_PID_parameters.vi"("error in"=w357, "Autofocus cluster"=w352, "PID gains"=w356, "queue MAIN"=w355) -> ("error out"=w354:errorcluster, "Autofocus cluster OUT"=w353:T2)
          }
        }
        n90 = case shown="False" w338 {
          tunnel: w310 -> [w362 w367]
          tunnel: w339 -> [w361 w366]
          tunnel: w340 -> [w359 w364]
          tunnel: [w358 w363] -> w343
          frame True {
            n91 = Multiply(x=w361, y=w362) -> (x*y=w360:dbl)
            n92 = Subtract(x=w359, y=w360) -> (x-y=w358:dbl)
          }
          frame False {
            n93 = Multiply(x=w366, y=w367) -> (x*y=w365:dbl)
            n94 = Add(x=w364, y=w365) -> (x+y=w363:dbl)
          }
        }
        n95 = Absolute Value(x=w310) -> (abs(x)=w312:dbl)
        n96 = Greater?(x=w312, y=0.1) -> (0:w309:bool)
        n97 = case shown="False" w309 {
          tunnel: w343 -> [_ w349]
          tunnel: w342 -> [_ w348]
          tunnel: [w345 w347] -> w323
          tunnel: w308 -> [w345 w346]
          frame False {
          }
          frame True {
            n98 = call "PIEZO_single_write_position.vi"("handle"=w348, "error in"=w346, "Zposition setpoint"=w349) -> ("error out"=w347:errorcluster)  [unwired: 2 in]
          }
        }
        n99 = call "PIEZO_read_position.vi"("MCL Handle"=w342, "Autofocus ON?"=TRUE, "error MCL in"=w323, "Autofocus cluster"=w320) -> ("error MCL out"=w324:errorcluster, "Autofocus cluster OUT"=w334:T2)  [unwired: 4 in, 2 out]
      }
      frame "Piezo_stop_autofocus" {
        n100 = call "PIEZO_task_START.vi"("error in"=w371) -> ("error out"=w370:errorcluster)
        n101 = Flush Queue(queue=w378, error in (no error)=w370) -> (error out=w369:errorcluster)  [unwired: 2 out]
        n102 = call "PIEZO_task_DONE.vi"("error in"=w369) -> ("error out"=w368:errorcluster)
      }
      frame "Piezo_init_autofocus_merFISH_TL" {
        w386 = 0 ("iteration")
        n103 = call "PIEZO_task_START.vi"("error in"=w408) -> ("error out"=w401:errorcluster)
        n104 = Unbundle By Name(w407) -> ("Ref channel"=w391:bool, "dimension size"=w398:i32)
        n105 = Flush Queue(queue=w404, error in (no error)=w401) -> (error out=w402:errorcluster)  [unwired: 2 out]
        n106 = Variant To Data(error in=w402, type=T5 {"PID gains"={"proportional gain (Kc)"=0.0, "integral time (Ti, min)"=0.0, "derivative time (Td, min)"=0.0}, "QPD ref"={"X"=0.0, "Y"=0.0, "SUM"=0.0, "count"=0}} ("output cluster"), Variant=w403) -> (data=w393:T5, error out=w397:errorcluster)
        n107 = Unbundle By Name(w393) -> ("PID gains"=w392:T8, "QPD ref"=w380:T9)
        n108 = case shown="True" w391 {
          tunnel: [w411 w413] -> w390
          tunnel: w380 -> [w412 w414]
          frame True {
            n109 = Unbundle By Name(w412) -> ("X"=w411:sgl)
          }
          frame False {
            n110 = Unbundle By Name(w414) -> ("Y"=w413:sgl)
          }
        }
        n111 = for {
          N: w398 -> [_]
          tunnel: [w417] -> w384 mode=indexing
          tunnel: w397 -> [w416]
          tunnel: [w416] -> w399
          i -> [w419]
          n112 = To Double Precision Float(number=w419) -> (double precision float=w415:dbl)
          n113 = Divide(x=w415, y=10.0) -> (x/y=w417:dbl)
        }
        n114 = Initialize Array(0.0 ("element"), w398) -> (w383:dbl[])
        n115 = call "PIEZO_read_position.vi"("MCL Handle"=w396, "error MCL in"=w399) -> ("error MCL out"=w388:errorcluster, "Z piezo"=w385:dbl)  [unwired: 6 in, 2 out]
        n116 = call "PIEZO_task_DONE.vi"("error in"=w388) -> ("error out"=w389:errorcluster)
        n117 = Bundle By Name(cluster=w407, "i IR lost"=w386, "iteration"=w386, "Switch"=FALSE, "Autocalibration"=FALSE, "PID gains"=w392, "Setpoint"=w390, "Y_derivation"=w383, "Derivation array"=w383, "X_derivation"=w384, "z0"=w385) -> (w409:T2)
      }
      frame "Piezo_autofocus_merFISH_TL" {
        n118 = Unbundle By Name(w432) -> ("z0"=w438:dbl, "Slope"=w437:dbl, "Switch"=w436:bool, "iteration"=w423:i32, "Setpoint"=w439:dbl, "PID gains"=w440:T8, "Ref channel"=w425:bool, "i IR lost"=w424:i32)
        n119 = call "AUTOFOCUS_read_QPD_signal_autofocus.vi"("error in"=w421, "i IR lost"=w424, "channel"=w425) -> ("error out"=w420:errorcluster, "IR lost?"=w430:bool, "i IR lost OUT"=w426:i32, "QPD"=w427:dbl)  [unwired: 2 in, 1 out]
        n120 = case shown="False" w430 {
          tunnel: [T1 {"variant"=variant, "Instruction"=enum."Piezo_autofocus_merFISH_TL"} ("Q_MCL_Piezo") T1 {"variant"=variant, "Instruction"=enum."Piezo_read_z"} ("Q_MCL_Piezo")] -> w441
          tunnel: w440 -> [w474 _]
          tunnel: w439 -> [w452 _]
          tunnel: w427 -> [w453 _]
          tunnel: w429 -> [w470 _]
          tunnel: w438 -> [w469 _]
          tunnel: w437 -> [w468 _]
          tunnel: w436 -> [w467 _]
          tunnel: [cluster{"z positions":dbl[], "z0":dbl} {"z positions"=[], "z0"=0.0} ("ramp cluster") cluster{"z positions":dbl[], "z0":dbl} {"z positions"=[], "z0"=0.0} ("ramp cluster")] -> w435
          tunnel: w423 -> [w443 _]
          tunnel: [w464 w487] -> w433
          tunnel: w432 -> [w460 w491]
          tunnel: w420 -> [w462 w493]
          tunnel: [w442 w491] -> w431
          tunnel: w429 -> [w461 _]
          tunnel: w428 -> [_ w488]
          tunnel: w426 -> [w459 _]
          tunnel: w423 -> [w454 _]
          frame False {
            n121 = Subtract(x=w452, y=w453) -> (x-y=w451:dbl)
            n122 = Less?(x=w454, y=20) -> (x < y?=w455:bool)
            n123 = Absolute Value(x=w451) -> (abs(x)=w448:dbl)
            n124 = call <vilib>:"PID Autotuning.vi"("reinitialize? (F)"=w455, "dt (s)"=1.0, "PID gains"=w474, "process variable"=w453, "setpoint"=w452) -> ("output"=w473:dbl)  [unwired: 3 in, 3 out]
            n125 = case shown="False" w467 {
              tunnel: w473 -> [w480 w485]
              tunnel: w468 -> [w479 w484]
              tunnel: w469 -> [w477 w482]
              tunnel: [w476 w481] -> w472
              frame True {
                n126 = Multiply(x=w479, y=w480) -> (x*y=w478:dbl)
                n127 = Subtract(x=w477, y=w478) -> (x-y=w476:dbl)
              }
              frame False {
                n128 = Multiply(x=w484, y=w485) -> (x*y=w483:dbl)
                n129 = Add(x=w482, y=w483) -> (x+y=w481:dbl)
              }
            }
            n130 = call "PIEZO_single_write_position.vi"("handle"=w470, "error in"=w462, "Zposition setpoint"=w472) -> ("error out"=w471:errorcluster)  [unwired: 2 in]
            n131 = Bundle By Name(cluster=w460, "i IR lost"=w459) -> (w457:T2)
            n132 = call "PIEZO_read_position.vi"("MCL Handle"=w461, "Autofocus ON?"=TRUE, "error MCL in"=w471, "Autofocus cluster"=w457) -> ("error MCL out"=w464:errorcluster, "Autofocus cluster OUT"=w442:T2, "Stable?"=w449:bool)  [unwired: 4 in, 1 out]
            n133 = Less?(x=w448, y=0.005) -> (x < y?=w446:bool)
            n134 = Greater?(x=w443, y=20) -> (0:w450:bool)
            n135 = Build Array(w450, w446, w449) -> (w445:bool[])
            n136 = And Array Elements(Boolean array=w445) -> (logical AND=w444:bool)
            n137 = global write "Global_MCL_piezo.vi" "Autofocus stable"(w444) -> ()
          }
          frame True {
            n138 = flat-sequence {
              tunnel: w493 -> [w494]
              tunnel: [w494] -> w489
              frame #0 {
                n139 = global write "Global_MCL_piezo.vi" "Autofocus lost"(TRUE ("Autofocus lost")) -> ()
              }
            }
            n140 = property class="Bool (strict)"(reference=w488, error in=w489, "Value"=TRUE) -> (error out=w487:errorcluster)  [unwired: 1 out]
          }
        }
      }
      frame "Piezo_autofocus_lost" {
        n141 = call "PIEZO_task_START.vi"("error in"=w512) -> ("error out"=w511:errorcluster)
        n142 = call "PIEZO_read_position.vi"("MCL Handle"=w499, "Autofocus ON?"=FALSE, "error MCL in"=w511) -> ("error MCL out"=w502:errorcluster, "Z piezo"=w500:dbl)  [unwired: 5 in, 2 out]
        n143 = In Range and Coerce(upper limit=70.0, x=w500, lower limit=10.0) -> (In Range?=w503:bool)  [unwired: 1 out]
        n144 = case shown="False" w503 {
          tunnel: w502 -> [w516 w527]
          tunnel: [w514 w527] -> w501
          tunnel: w500 -> [w518 _]
          tunnel: w499 -> [w513 _]
          frame False {
            n145 = Greater?(x=10.0, y=w518) -> (0:w515:bool)
            n146 = case shown="False" w515 {
              tunnel: w516 -> [w522 w526]
              tunnel: [w521 w525] -> w514
              tunnel: w513 -> [w520 w524]
              frame True {
                n147 = call "PIEZO_single_write_position.vi"("handle"=w520, "error in"=w522, "Zposition setpoint"=20.0) -> ("error out"=w521:errorcluster)  [unwired: 2 in]
              }
              frame False {
                n148 = call "PIEZO_single_write_position.vi"("handle"=w524, "error in"=w526, "Zposition setpoint"=60.0) -> ("error out"=w525:errorcluster)  [unwired: 2 in]
              }
            }
          }
          frame True {
          }
        }
        n149 = call "PIEZO_task_DONE.vi"("error in"=w501) -> ("error out"=w498:errorcluster)
      }
      frame "Piezo_resume_autofocus_merFISH_TL" {
        n150 = call "PIEZO_task_START.vi"("error in"=w553) -> ("error out"=w529:errorcluster)
        n151 = Bundle By Name(cluster=w547, "iteration"=0) -> (w545:T2)
        n152 = Flush Queue(queue=w528, error in (no error)=w529) -> (error out=w530:errorcluster)  [unwired: 2 out]
        n153 = call "PIEZO_read_position.vi"("MCL Handle"=w542, "error MCL in"=w530) -> ("error MCL out"=w538:errorcluster, "Z piezo"=w541:dbl)  [unwired: 6 in, 2 out]
        n154 = Unbundle By Name(w545) -> ("Slope"=w552:dbl, "Switch"=w551:bool, "Setpoint"=w550:dbl, "PID gains"=w549:T8, "Ref channel"=w539:bool)
        n155 = while {
          tunnel: w549 -> [w594]
          tunnel: w550 -> [w593]
          tunnel: w542 -> [w589]
          tunnel: w552 -> [w587]
          tunnel: w551 -> [w586]
          tunnel: w542 -> [w584]
          shift-right: [w573] -> w537
          shift-left: w538 -> [w572]
          shift-right: [w582] -> w532
          shift-left: w545 -> [w562]
          shift-right: [w577] -> _
          shift-left: w541 -> [w576]
          tunnel: w539 -> [w570]
          tunnel: [w566] -> w534
          i -> [w581]
          stop <- w574 stop-if-true
          n156 = Unbundle By Name(w562) -> ("i IR lost"=w561:i32)
          n157 = call "AUTOFOCUS_read_QPD_signal_autofocus.vi"("error in"=w572, "i IR lost"=w561, "channel"=w570) -> ("error out"=w571:errorcluster, "IR lost?"=w568:bool, "i IR lost OUT"=w564:i32, "QPD"=w565:dbl)  [unwired: 2 in, 1 out]
          n158 = global write "Global_MCL_piezo.vi" "Autofocus lost"(w568) -> ()
          n159 = Bundle By Name(cluster=w562, "i IR lost"=w564) -> (w563:T2)
          n160 = call <vilib>:"PID Autotuning.vi"("reinitialize? (F)"=TRUE, "dt (s)"=1.0, "PID gains"=w594, "process variable"=w565, "setpoint"=w593) -> ("output"=w592:dbl)  [unwired: 3 in, 3 out]
          n161 = case shown="False" w586 {
            tunnel: w592 -> [w599 w604]
            tunnel: w587 -> [w598 w603]
            tunnel: w576 -> [w596 w601]
            tunnel: [w595 w600] -> w591
            frame True {
              n162 = Multiply(x=w598, y=w599) -> (x*y=w597:dbl)
              n163 = Subtract(x=w596, y=w597) -> (x-y=w595:dbl)
            }
            frame False {
              n164 = Multiply(x=w603, y=w604) -> (x*y=w602:dbl)
              n165 = Add(x=w601, y=w602) -> (x+y=w600:dbl)
            }
          }
          n166 = call "PIEZO_single_write_position.vi"("handle"=w589, "error in"=w571, "Zposition setpoint"=w591) -> ("error out"=w590:errorcluster)  [unwired: 2 in]
          n167 = call "PIEZO_read_position.vi"("MCL Handle"=w584, "Autofocus ON?"=TRUE, "error MCL in"=w590, "Autofocus cluster"=w563) -> ("error MCL out"=w573:errorcluster, "Autofocus cluster OUT"=w582:T2, "Z piezo"=w577:dbl, "Stable?"=w578:bool)  [unwired: 4 in]
          n168 = global read "Global_ABORT.vi" "ABORT"() -> (w575:bool)
          n169 = Not(x=w568) -> (.not. x?=w567:bool)
          n170 = Greater?(x=w581, y=20) -> (0:w579:bool)
          n171 = And(x=w579, y=w578) -> (x .and. y?=w569:bool)
          n172 = Or(x=w575, y=w569) -> (x .or. y?=w574:bool)
          n173 = And(x=w567, y=w569) -> (x .and. y?=w566:bool)
        }
        n174 = case shown="True" w534 {
          tunnel: w537 -> [w554 w558]
          tunnel: [w554 w557] -> w536
          tunnel: w535 -> [_ w555]
          frame False {
          }
          frame True {
            n175 = property class="Bool (strict)"(reference=w555, error in=w558, "Value"=FALSE) -> (error out=w557:errorcluster)  [unwired: 1 out]
          }
        }
        n176 = case shown="True" w534 {
          tunnel: [T1 {"variant"=variant, "Instruction"=enum."Piezo_read_z"} ("Q_MCL_Piezo") T1 {"variant"=variant, "Instruction"=enum."Piezo_autofocus_merFISH_TL"} ("Q_MCL_Piezo")] -> w544
          frame False {
          }
          frame True {
          }
        }
        n177 = Bundle By Name(cluster=w532, "iteration"=0) -> (w531:T2)
        n178 = call "PIEZO_task_DONE.vi"("error in"=w536) -> ("error out"=w540:errorcluster)
      }
      frame "Piezo_check_z_position_merFISH_TL" {
        n179 = call "PIEZO_task_START.vi"("error in"=w616) -> ("error out"=w606:errorcluster)
        n180 = call "PIEZO_read_position.vi"("MCL Handle"=w613, "error MCL in"=w606) -> ("error MCL out"=w609:errorcluster, "Z piezo"=w608:dbl)  [unwired: 6 in, 2 out]
        n181 = global write "Global_MCL_piezo.vi" "z"(w608) -> ()
        n182 = call "PIEZO_task_DONE.vi"("error in"=w609) -> ("error out"=w612:errorcluster)
        n183 = case shown="True" w605 {
          tunnel: [T1 {"variant"=variant, "Instruction"=enum."Piezo_idle"} ("Q_MCL_Piezo") T1 {"variant"=variant, "Instruction"=enum."Piezo_autofocus_merFISH_TL"} ("Q_MCL_Piezo")] -> w610
          frame False {
          }
          frame True {
          }
        }
      }
      frame "Piezo_stop_autofocus_merFISH_TL" {
        n184 = call "PIEZO_task_START.vi"("error in"=w621) -> ("error out"=w623:errorcluster)
        n185 = Flush Queue(queue=w619, error in (no error)=w623) -> (error out=w622:errorcluster)  [unwired: 2 out]
        n186 = call "PIEZO_task_DONE.vi"("error in"=w622) -> ("error out"=w620:errorcluster)
      }
      frame "Piezo_init_ramp" {
        n187 = call "Piezo_task_START.vi"("error in"=w646) -> ("error out"=w634:errorcluster)
        n188 = Flush Queue(queue=w632, error in (no error)=w634) -> (error out=w633:errorcluster)  [unwired: 2 out]
        n189 = call "PIEZO_read_position.vi"("MCL Handle"=w645, "error MCL in"=w633) -> ("error MCL out"=w641:errorcluster, "Z piezo"=w637:dbl)  [unwired: 6 in, 2 out]
        n190 = Bundle By Name(cluster=w639, "z0"=w637) -> (w638:cluster{"z positions":dbl[], "z0":dbl})
        n191 = global write "Global_MCL_piezo.vi" "z"(w637) -> ()
        n192 = case shown="No Error" w641 {
          selector: w641 -> [w648 w650]
          tunnel: [w648 w650] -> w640
          frame Error {
            n193 = global write "Global_MCL_piezo.vi" "Piezo ready"(FALSE ("Piezo ready")) -> ()
          }
          frame No Error {
            n194 = global write "Global_MCL_piezo.vi" "Piezo ready"(TRUE ("Piezo ready")) -> ()
          }
        }
        n195 = call "Piezo_task_DONE.vi"("error in"=w640) -> ("error out"=w643:errorcluster)
      }
      frame "Piezo_move_z_ramp" {
        n196 = call "PIEZO_task_START.vi"("error in"=w674) -> ("error out"=w672:errorcluster)
        n197 = Variant To Data(error in=w672, type=cluster{"i":i32, "N":i32, "z":dbl} {"i"=0, "N"=0, "z"=0.0} ("output cluster"), Variant=w673) -> (data=w664:cluster{"i":i32, "N":i32, "z":dbl}, error out=w671:errorcluster)
        n198 = Unbundle By Name(w664) -> ("N"=w660:i32, "i"=w658:i32, "z"=w663:dbl)
        n199 = call "PIEZO_single_write_position.vi"("handle"=w669, "error in"=w671, "Zposition setpoint"=w663) -> ("error out"=w670:errorcluster)  [unwired: 2 in]
        n200 = Unbundle By Name(w656) -> ("z positions"=w657:dbl[])
        n201 = Equal To 0?(x=w658) -> (x = 0?=w662:bool)
        n202 = call "PIEZO_read_position.vi"("MCL Handle"=w669, "error MCL in"=w670) -> ("error MCL out"=w668:errorcluster, "Z piezo"=w659:dbl)  [unwired: 6 in, 2 out]
        n203 = case shown="False" w662 {
          tunnel: w660 -> [w679 _]
          tunnel: w657 -> [_ w681]
          tunnel: w659 -> [w676 w683]
          tunnel: w658 -> [w677 w684]
          tunnel: [w675 w682] -> w655
          frame True {
            n204 = Initialize Array(0.0 ("element"), w679) -> (w678:dbl[])
            n205 = Replace Array Subset(array=w678, new element=w676, index=w677) -> (w675:dbl[])
          }
          frame False {
            n206 = Replace Array Subset(array=w681, new element=w683, index=w684) -> (w682:dbl[])
          }
        }
        n207 = call "PIEZO_task_DONE.vi"("error in"=w668) -> ("error out"=w667:errorcluster)
        n208 = Bundle By Name(cluster=w656, "z positions"=w655) -> (w654:cluster{"z positions":dbl[], "z0":dbl})
      }
      frame "Piezo_close_ramp" {
        n209 = call "Piezo_task_START.vi"("error in"=w706) -> ("error out"=w701:errorcluster)
        n210 = global read "Global_ABORT.vi" "ABORT"() -> (w698:bool)
        n211 = Unbundle By Name(w690) -> ("z0"=w693:dbl, "z positions"=w696:dbl[])
        n212 = Variant To Data(error in=w701, type=path "" ("Z_position_file path"), Variant=w702) -> (data=w697:path, error out=w699:errorcluster)
        n213 = case shown="False" w698 {
          tunnel: w699 -> [w710 w711]
          tunnel: w697 -> [w709 _]
          tunnel: w696 -> [w708 _]
          tunnel: [w707 w711] -> w694
          frame False {
            n214 = call "RAMP_save_Z_scan_positions.vi"("error in"=w710, "base path"=w709, "Z array"=w708) -> ("error out"=w707:errorcluster)  [unwired: 1 in]
          }
          frame True {
          }
        }
        n215 = call "PIEZO_single_write_position.vi"("handle"=w692, "error in"=w694, "Zposition setpoint"=w693) -> ("error out"=w695:errorcluster)  [unwired: 2 in]
        n216 = call "PIEZO_read_position.vi"("MCL Handle"=w692, "error MCL in"=w695) -> ("error MCL out"=w691:errorcluster)  [unwired: 6 in, 3 out]
        n217 = call "Piezo_task_DONE.vi"("error in"=w691) -> ("error out"=w704:errorcluster)
        n218 = Bundle By Name(cluster=w690, "z positions"=dbl[] []) -> (w689:cluster{"z positions":dbl[], "z0":dbl})
      }
      frame "Piezo_close_merFISH" {
        n219 = call "PIEZO_task_START.vi"("error in"=w718) -> ("error out"=w717:errorcluster)
        n220 = Flush Queue(queue=w723, error in (no error)=w717) -> (error out=w715:errorcluster)  [unwired: 2 out]
        n221 = flat-sequence {
          tunnel: w715 -> [w726]
          tunnel: [w726] -> w714
          frame #0 {
            w725 = FALSE
            n222 = global write "Global_MCL_piezo.vi" "Autofocus stable"(w725) -> ()
            n223 = global write "Global_MCL_piezo.vi" "Piezo ready"(w725) -> ()
          }
        }
        n224 = call "PIEZO_task_DONE.vi"("error in"=w714) -> ("error out"=w716:errorcluster)
      }
      frame "Piezo_stop" {
        n225 = Flush Queue(queue=w731, error in (no error)=w739) -> (error out=w732:errorcluster)  [unwired: 2 out]
        n226 = call "PIEZO_task_START.vi"("error in"=w732) -> ("error out"=w730:errorcluster)
        n227 = dll-call lib="C:/Program Files/National Instruments/LabVIEW 2015/user.lib/Madlib.dll" fn="MCL_ReleaseAllHandles"(error in=w730) -> (error out=w738:errorcluster)  [unwired: 3 in, 1 out]
        n228 = call-poly <vilib>:"Close Input Device.vi"("error in (no error)"=w738, "device ID"=w737) -> ("error out"=w736:errorcluster)  [unwired: 8 in]
        n229 = call "PIEZO_task_DONE.vi"("error in"=w736) -> ("error out"=w729:errorcluster)
      }
    }
    n230 = global read "Global_MAIN.vi" "Stop main vi"() -> (w54:bool)
    n231 = To Variant(anything=w39) -> (Variant=w41:variant)
    n232 = Wait (ms)(milliseconds to wait=w32) -> ()  [unwired: 1 out]
    n233 = Bundle By Name(cluster=T1 {"variant"=variant, "Instruction"=enum."Piezo_error"} ("Q_MCL_Piezo"), "variant"=w41) -> (w38:T1)
    n234 = case shown="No Error" w39 {
      selector: w39 -> [w56 _]
      tunnel: w49 -> [w55 _]
      tunnel: [w59 w63] -> w48
      tunnel: [w58 w62] -> w47
      tunnel: w26 -> [w57 w61]
      tunnel: w38 -> [_ w60]
      frame No Error {
        n235 = Enqueue Element(queue=w57, element=w55, error in (no error)=w56) -> (queue out=w59:refnum<queue>, error out=w58:errorcluster)  [unwired: 1 in, 1 out]
      }
      frame Error {
        n236 = Enqueue Element(queue=w61, element=w60) -> (queue out=w63:refnum<queue>, error out=w62:errorcluster)  [unwired: 2 in, 1 out]
      }
    }
  }
  n237 = Release Queue(queue=w19, error in (no error)=w18) -> ()  [unwired: 1 in, 3 out]
